vi "BatterySim_CalculateDefaultBatteryLoadedVoltage.vi"(11 "Currents":dbl[](array[numeric])) -> (3 "Voltage":dbl)   [LabVIEW 2019, in "Trajectory_Library.lvlib"]
doc: "Calculate the loaded battery voltage. This function assumes a nominal voltage of 12v and a resistance of 20 milliohms (0.020 ohms)\n \nInputs:\n - currents -- An array of currents drawn from the battery.\n\nOutputs:\n - Voltage -- The battery's voltage under load."
uses:
  Trajectory_Library.lvlib
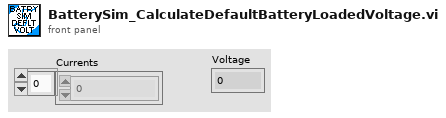
[diagram p1: front panel]
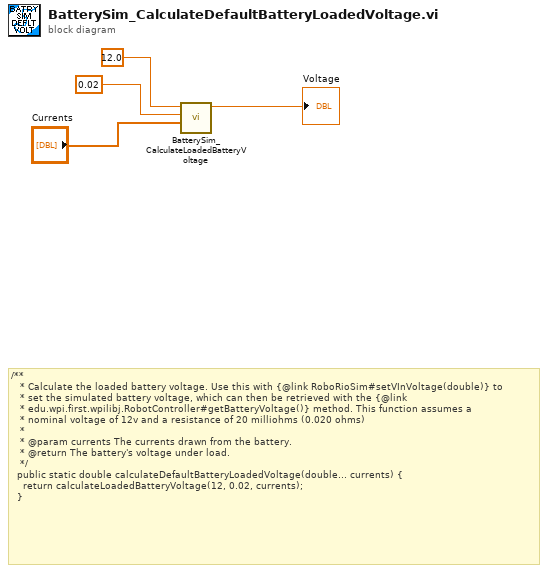
[diagram p0: block diagram]
diagram:
  # "/**\n   * Calculate the loaded battery voltage. Use this with {@link RoboRioSim#setVInVoltage(double)} to\n   * set the simulated battery voltage, which can then be retrieved with the {@link\n   * edu.wpi.first.wpilibj.RobotController#getBatteryVoltage()} method. This function assumes a\n   * nominal voltage of 12v and a resistance of 20 milliohms (0.020 ohms)\n   *\n   * @param currents The currents drawn from the battery.\n   * @return The battery's voltage under load.\n   */\n  public static double calculateDefaultBatteryLoadedVoltage(double... currents) {\n    return calculateLoadedBatteryVoltage(12, 0.02, currents);\n  }"
  n1 = call "BatterySim_CalculateLoadedBatteryVoltage.vi"("Currents"="Currents", "Resistance_Ohms"=0.02, "NominalVoltage"=12.0) -> ("Voltage"=→"Voltage":dbl)  [unwired: 8 in]
